vi "Read Command Processor Status.vi"(8 "error in (no error)":errorcluster, 11 "Command Processor in":refnum<class "Command Processor.lvclass">) -> (0 "error out":errorcluster, 2 "Command Processor Status":T1, 3 "Command Processor out":refnum<class "Command Processor.lvclass">)   [LabVIEW 2013, in "Robot Actors.lvlib" / "Command Processor.lvlib" / "Command Processor.lvclass"]
uses:
  Command Processor.lvclass
  Command Processor Status.ctl
  Command/Command Class/Command Status.ctl
  Command/Command Class/Command States.ctl
  Command Processor States.ctl
  Command Processor.lvclass/Command Processor.ctl
  Command/Command Class/Command.lvclass
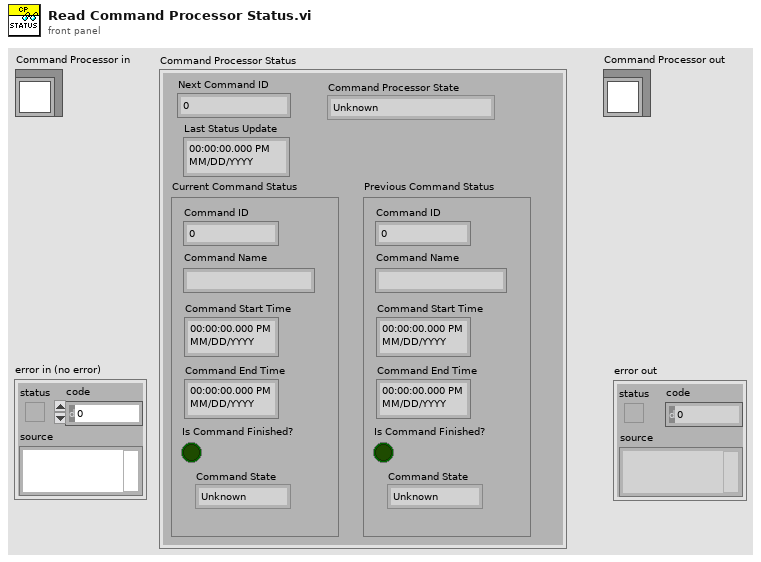
[diagram p1: front panel]
types:
  T1 = typedef "Robot Actors.lvlib/Command Processor.lvlib/Command Processor.lvclass/Command Processor Status.ctl" = cluster{"Next Command ID":dbl, "Current Command Status":T2, "Previous Command Status ":T2, "Command Processor State":T4, "Last Status Update":timestamp}
  T2 = typedef "Robot Actors.lvlib/Command.lvlib/Command.lvclass/Command Status.ctl" = cluster{"Command Name":string, "Command Start Time":timestamp, "Command End Time":timestamp, "Is Command Finished?":bool, "Command ID":dbl, "Command State":T3}
  T3 = typedef "Robot Actors.lvlib/Command.lvlib/Command.lvclass/Command States.ctl" = enum16{"Unknown", "Started", "Stopped", "Finished"}
  T4 = typedef "Robot Actors.lvlib/Command Processor.lvlib/Command Processor.lvclass/Command Processor States.ctl" = enum16{"Unknown", "No Command", "Running Command"}
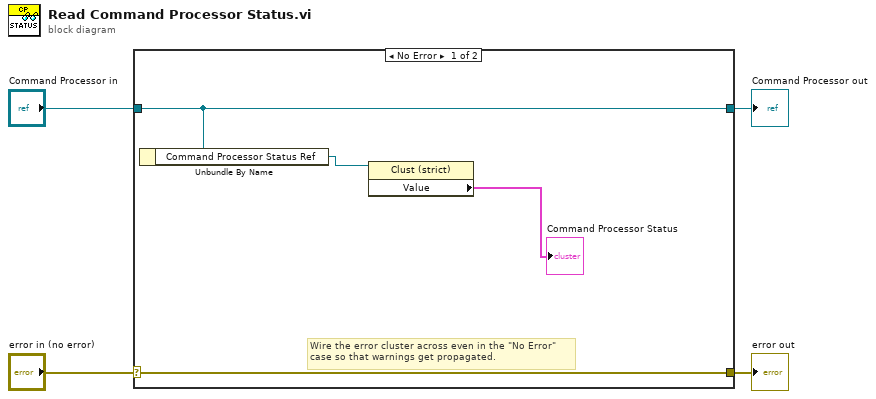
[diagram p0: block diagram]
diagram:
  n1 = case shown="No Error" "error in (no error)" {
    selector: "error in (no error)" -> [w8 w10]
    tunnel: [w8 w10] -> w3
    tunnel: [w7 w9] -> w1
    tunnel: "Command Processor in" -> [w7 w9]
    frame No Error {
      # "Wire the error cluster across even in the \"No Error\"\ncase so that warnings get propagated."
      n2 = Unbundle By Name(w7) -> ("Command Processor Status Ref"=w6:refnum<vi>)
      n3 = property class="Clust (strict)"(reference=w6) -> ("Value"=→"Command Processor Status":T1)  [unwired: 1 in, 2 out]
    }
    frame Error {
    }
  }
  "error out" <- w3
  "Command Processor out" <- w1
